vi "GetGUID.vi"(8 "error in (no error)":errorcluster) -> (0 "error out":errorcluster, 3 "GUID":string)   [LabVIEW 2016, in "SRP.lvlib"]
uses:
  <vilib>/addons/InsightCM/SRP/SRP.lvlib
  <vilib>/addons/InsightCM/SRP/libraries/win32Urelease/brsrp.dll
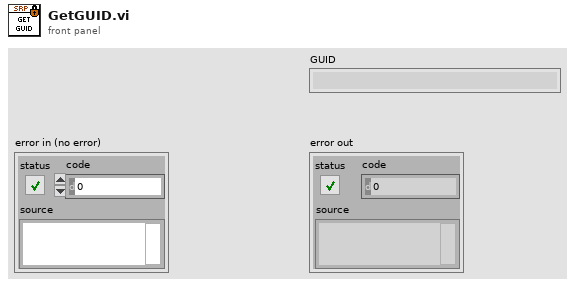
[diagram p1: front panel]
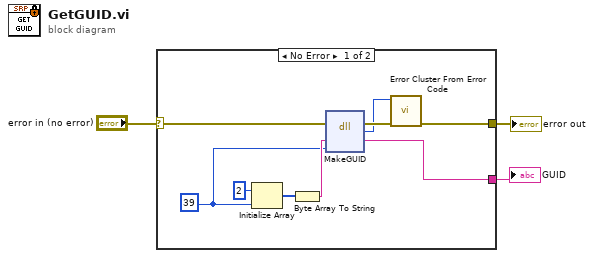
[diagram p0: block diagram]
diagram:
  n1 = case shown="No Error" "error in (no error)" {
    selector: "error in (no error)" -> [w11 w13]
    tunnel: [w12 _] -> w3
    tunnel: [w5 w13] -> w2
    frame No Error {
      w4 = 39 ("length")
      n2 = Initialize Array(u8 2 ("dimension size"), w4) -> (w8:u8[])
      n3 = Byte Array To String(unsigned byte array=w8) -> (string=w7:string)
      n4 = dll-call lib="C:/Program Files (x86)/National Instruments/LabVIEW 2016/vi.lib/addons/InsightCM/SRP/libraries/win32Urelease/brsrp.*" fn="MakeGUID"(error in=w11, "guid"=w7, "length"=w4) -> (error out=w10:errorcluster, "return type"=w6:i32, "guid"=w12:string)  [unwired: 3 in, 1 out]
      n5 = call <vilib>:"Error Cluster From Error Code.vi"("error in (no error)"=w10, "error code (0)"=w6) -> ("error out"=w5:errorcluster)  [unwired: 7 in]
    }
    frame Error {
    }
  }
  "error out" <- w2
  "GUID" <- w3
